vi "1D Array to String - Performant.vi"(7 "delimiter (Tab)":string, 10 "Array of Strings":string[](array[string])) -> (1 "delimited string":string)   [LabVIEW 2009]
doc: "Converts 1D Array of strings to a delimited string"
panel:
  # "[OpenG VI Tags] ***Do Not Remove***"
  # "1D Array to String.vi\n\nConverts 1D Array of strings to a delimited string.\n\nPlease visit http://www.OpenG.org to learn about the\nOpen Source LabVIEW software movement.\n\nNOTICE -- YOU MUST LEAVE THIS NOTICE IN PLACE.  PER THE TERMS OF THE LICENSE BELOW, YOU MAY SUBLICENSE THIS SOFTWARE \nIN ANY WAY THAT DOES NOT CONFLICT WITH THIS LICENSE.\n\n### BSD License (http://www.opensource.org/licenses/bsd-license.php) Begin ###\n \nCopyright (c) 2002, Jim Kring <jim@jimkring.com>\n\nAll rights reserved.\n\nRedistribution and use in source and binary forms, with or without modification, are permitted provided that the following conditions are met:\n\n    * Redistributions of source code must retain the above copyright notice, this list of conditions and the following disclaimer.\n    * Redistributions in binary form must reproduce the above copyright notice, this list of conditions and the following disclaimer in the \n       documentation and/or other materials provided with the distribution.\n    * Neither the name of SciWare, James Kring, Inc., nor the names of its contributors may be used to endorse or promote products derived \n       from this software without specific prior written permission.\n\nTHIS SOFTWARE IS PROVIDED BY THE COPYRIGHT HOLDERS AND CONTRIBUTORS \"AS IS\" AND ANY EXPRESS OR IMPLIED WARRANTIES, \nINCLUDING, BUT NOT LIMITED TO, THE IMPLIED WARRANTIES OF MERCHANTABILITY AND FITNESS FOR A PARTICULAR PURPOSE ARE \nDISCLAIMED. IN NO EVENT SHALL THE COPYRIGHT OWNER OR CONTRIBUTORS BE LIABLE FOR ANY DIRECT, INDIRECT, INCIDENTAL,\n SPECIAL, EXEMPLARY, OR CONSEQUENTIAL DAMAGES (INCLUDING, BUT NOT LIMITED TO, PROCUREMENT OF SUBSTITUTE GOODS OR \nSERVICES; LOSS OF USE, DATA, OR PROFITS; OR BUSINESS INTERRUPTION) HOWEVER CAUSED AND ON ANY THEORY OF LIABILITY, \nWHETHER IN CONTRACT, STRICT LIABILITY, OR TORT (INCLUDING NEGLIGENCE OR OTHERWISE) ARISING IN ANY WAY OUT OF THE USE \nOF THIS SOFTWARE, EVEN IF ADVISED OF THE POSSIBILITY OF SUCH DAMAGE.\n\n### BSD License End ###"
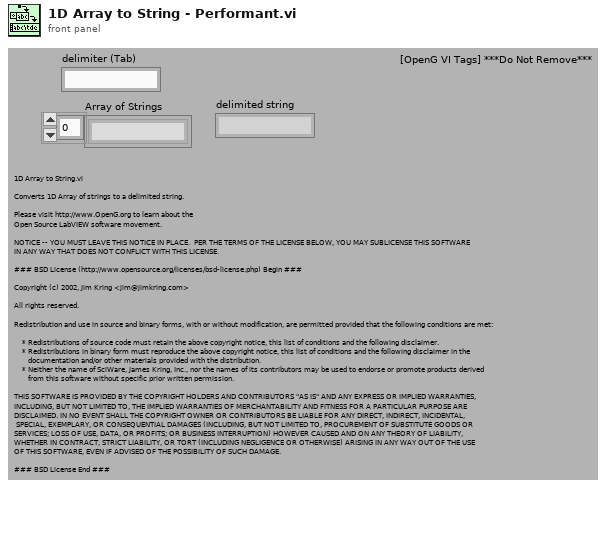
[diagram p1: front panel]
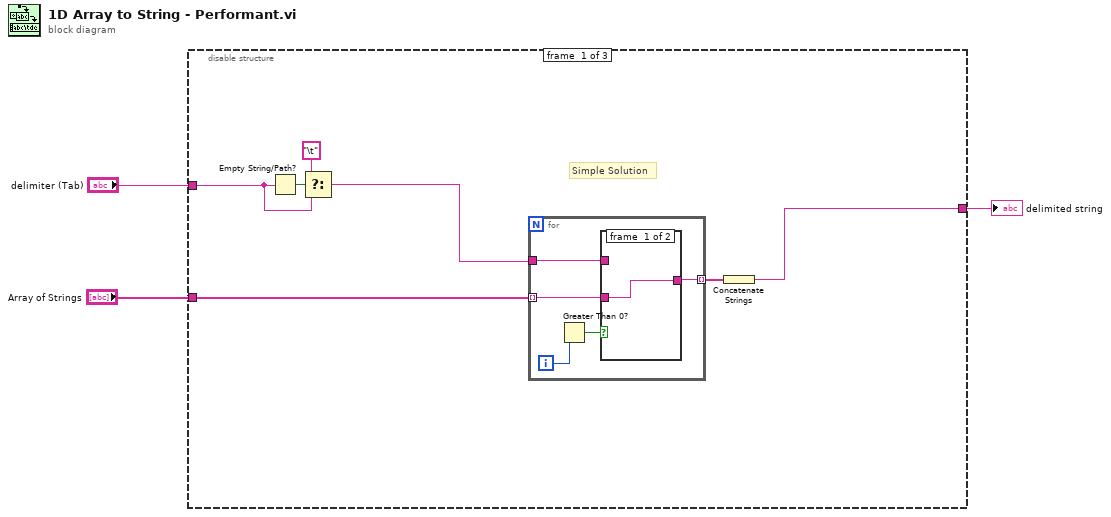
[diagram p0: block diagram]
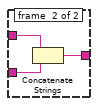
[diagram p2: hidden frame]
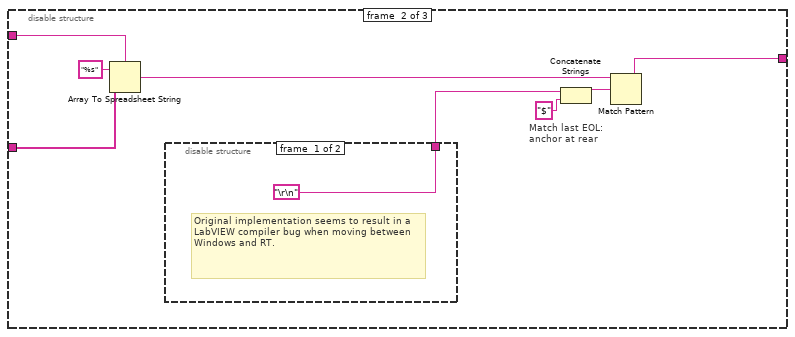
[diagram p3: hidden frame]
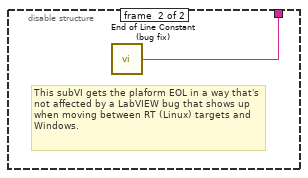
[diagram p4: hidden frame]
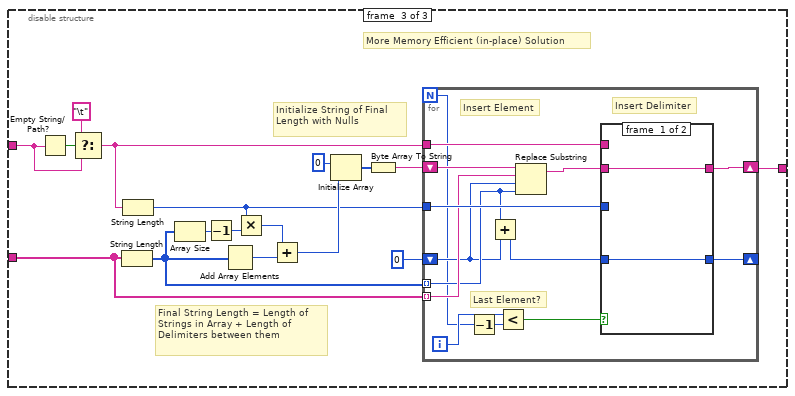
[diagram p5: hidden frame]
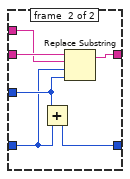
[diagram p6: hidden frame]
diagram:
  n1 = disable-structure shown="Disabled" {
    disable-tunnel: [w10 w21 w34] -> w3
    disable-tunnel: "Array of Strings" -> [w8 w22 w37]
    disable-tunnel: "delimiter (Tab)" -> [w4 w23 w31]
    frame #0 {
      # "Simple Solution"
      n2 = Empty String/Path?(string/path=w4) -> (empty?=w7:bool)
      n3 = Select(t="\t", s=w7, f=w4) -> (s? t:f=w5:string)
      n4 = for {
        tunnel: w8 -> [w12] mode=indexing
        tunnel: w5 -> [w13]
        tunnel: [w11] -> w9 mode=indexing
        i -> [w15]
        n5 = Greater Than 0?(x=w15) -> (x > 0?=w14:bool)
        n6 = case shown="True" w14 {
          tunnel: w13 -> [_ w19]
          tunnel: w12 -> [w16 w18]
          tunnel: [w16 w17] -> w11
          frame #0 {
          }
          frame #1 {
            n7 = Concatenate Strings(w19, w18) -> (w17:string)
          }
        }
      }
      n8 = Concatenate Strings(w9) -> (w10:string)
    }
    frame #1 {
      # "Match last EOL:\nanchor at rear"
      n9 = Array To Spreadsheet String(delimiter (Tab)=w23, array=w22, 3:"%s" ("format string")) -> (spreadsheet string=w24:string)
      n10 = disable-structure shown="Enabled" {
        disable-tunnel: ["\r\n" w29] -> w20
        frame #0 {
          # "Original implementation seems to result in a LabVIEW compiler bug when moving between Windows and RT."
        }
        frame #1 {
          # "This subVI gets the plaform EOL in a way that's not affected by a LabVIEW bug that shows up when moving between RT (Linux) targets and Windows."
          n11 = call "End of Line Constant (bug fix).vi"() -> ("Platform EOL"=w29:string)  [unwired: 5 in]
        }
      }
      n12 = Concatenate Strings(w20, "$" ("Substring")) -> (w25:string)
      n13 = Match Pattern(string=w24, regular expression=w25) -> (before substring=w21:string)  [unwired: 1 in, 3 out]
    }
    frame #2 {
      # "More Memory Efficient (in-place) Solution"
      # "Final String Length = Length of Strings in Array + Length of Delimiters between them"
      # "Initialize String of Final Length with Nulls"
      n14 = Empty String/Path?(string/path=w31) -> (empty?=w33:bool)
      n15 = Select(t="\t", s=w33, f=w31) -> (s? t:f=w30:string)
      n16 = String Length(string=w37) -> (length=w36:i32[])
      n17 = String Length(string=w30) -> (length=w35:i32)
      n18 = Array Size(array=w36) -> (size(s)=w46:i32)
      n19 = Decrement(x=w46) -> (x-1=w45:i32)
      n20 = Add Array Elements(numeric array=w36) -> (sum=w44:i32)
      n21 = Multiply(x=w35, y=w45) -> (x*y=w39:i32)
      n22 = Add(x=w39, y=w44) -> (x+y=w38:i32)
      n23 = Initialize Array(u8 0, w38) -> (w42:u8[])
      n24 = Byte Array To String(unsigned byte array=w42) -> (string=w41:string)
      n25 = for {
        N -> [w48]
        shift-right: [w54] -> w34
        shift-left: w41 -> [w50]
        shift-right: [w53] -> _
        shift-left: 0 -> [w51]
        tunnel: w37 -> [w57] mode=indexing
        tunnel: w36 -> [w56] mode=indexing
        tunnel: w35 -> [w58]
        tunnel: w30 -> [w59]
        i -> [w49]
        # "Insert Delimiter"
        # "Last Element?"
        # "Insert Element"
        n26 = Decrement(x=w48) -> (x-1=w47:i32)
        n27 = Add(x=w56, y=w51) -> (x+y=w52:i32)
        n28 = Less?(x=w49, y=w47) -> (x < y?=w60:bool)
        n29 = Replace Substring(2:w56, 3:w51, 4:w57, 5:w50) -> (1:w55:string)  [unwired: 1 out]
        n30 = case shown="True" w60 {
          tunnel: w55 -> [w62 w68]
          tunnel: w59 -> [_ w67]
          tunnel: w52 -> [w61 w65]
          tunnel: w58 -> [_ w66]
          tunnel: [w61 w64] -> w53
          tunnel: [w62 w63] -> w54
          frame #0 {
          }
          frame #1 {
            n31 = Add(x=w66, y=w65) -> (x+y=w64:i32)
            n32 = Replace Substring(2:w66, 3:w65, 4:w67, 5:w68) -> (1:w63:string)  [unwired: 1 out]
          }
        }
      }
    }
  }
  "delimited string" <- w3
